vi "全局停止（FG).vi"(7 "Default":bool, 8 "error in (no error)":errorcluster caption="错误输入（无错误）", 10 "Mode":enum16{"Init", "Set", "Get"}(ring)=enum."Get", 11 "Input":bool) -> (0 "error out":errorcluster caption="错误输出", 3 "Output":bool)   [LabVIEW 2012]
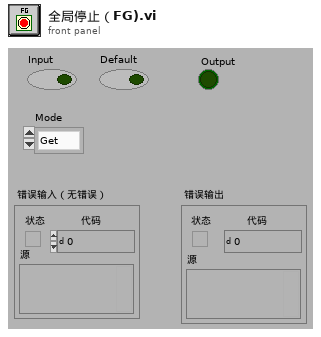
[diagram p1: front panel]
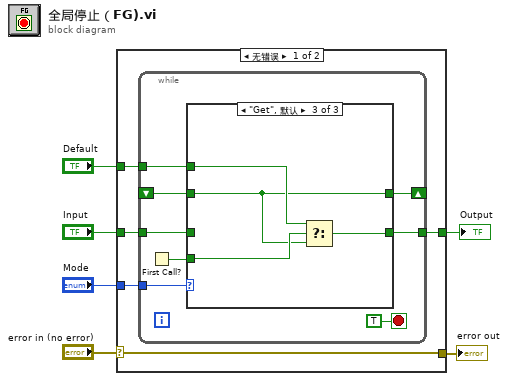
[diagram p0: block diagram]
diagram:
  n1 = case shown="无错误" "error in (no error)" {
    selector: "error in (no error)" -> [w7 w26]
    tunnel: [w7 w26] -> w1
    tunnel: "Mode" -> [w11 _]
    tunnel: "Input" -> [w10 _]
    tunnel: [w9 _] -> w5
    tunnel: "Default" -> [w8 _]
    frame No Error {
      n2 = while {
        shift-right: [w17] -> _
        shift-left: _ -> [w13]
        tunnel: w10 -> [w19]
        tunnel: [w18] -> w9
        tunnel: w8 -> [w16]
        tunnel: w11 -> [w15]
        stop <- TRUE stop-if-true
        n3 = First Call?() -> (First Call?: T/F=w14:bool)
        n4 = case shown="\"Get\", 默认" w15 {
          tunnel: w19 -> [_ w21 _]
          tunnel: [w20 w21 w23] -> w18
          tunnel: [w20 w21 w22] -> w17
          tunnel: w16 -> [w20 _ w24]
          tunnel: w14 -> [_ _ w25]
          tunnel: w13 -> [_ _ w22]
          frame "Init" {
          }
          frame "Set" {
          }
          frame "Get", Default {
            n5 = Select(t=w24, s=w25, f=w22) -> (s? t:f=w23:bool)
          }
        }
      }
    }
    frame Error {
    }
  }
  "error out" <- w1
  "Output" <- w5
